vi "Book Picture - p24_h2e.vi"() -> ()   [LabVIEW 2013]
uses:
  <vilib>/Analysis/baseanly.llb/Real A x B.vi
  <vilib>/Analysis/baseanly.llb/Real Inverse Matrix.vi
  <vilib>/Analysis/NI_AALBase.lvlib
panel:
  out "Y1":dbl=1.7320508075688776 format="%#_5g"
  out "X1":dbl=1.7320508075688776 format="%#_5g"
  # "Coodinate Reference System"
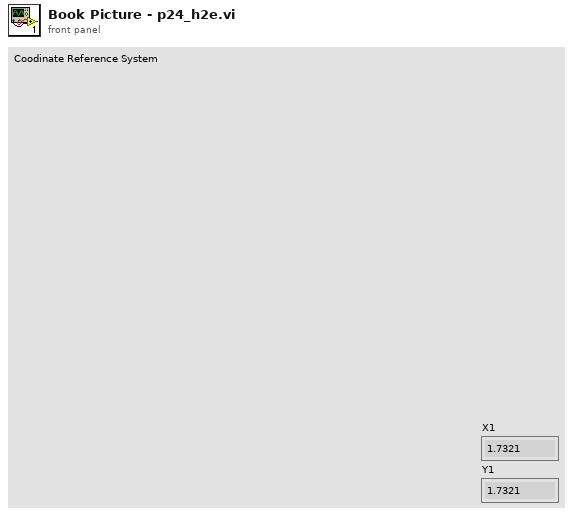
[diagram p1: front panel]
types:
  T1 = typedef "NI_Matrix.lvlib/RealMatrix.ctl" = dbl[][]
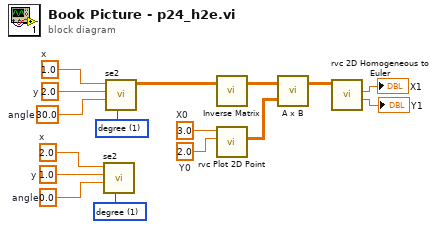
[diagram p0: block diagram]
diagram:
  w11 = 2.0  # Y0
  w12 = 3.0  # X0
  w3 = 0.0  # angle
  w2 = 1.0  # y
  w1 = 2.0  # x
  w4 = u16 1 items=["radians", "degree"] ("angle unit")
  w14 = 30.0  # angle
  w15 = 2.0  # y
  w16 = 1.0  # x
  w13 = u16 1 items=["radians", "degree"] ("angle unit")
  n1 = call "se2.vi"("angle unit"=w4, "theta"=w3, "y"=w2, "x"=w1) -> ()  [unwired: 6 in, 2 out]
  n2 = call "se2.vi"("angle unit"=w13, "theta"=w14, "y"=w15, "x"=w16) -> ("T"=w9:dbl[][])  [unwired: 6 in, 1 out]
  n3 = call-poly <vilib>:"Inverse Matrix.vi"("Input Matrix"=w9) -> ("Inverse Matrix"=w10:T1)  [unwired: 1 in, 1 out]
  n4 = call "rvc Plot 2D Point.vi"("Y"=w11, "X"=w12) -> ("Column vector"=w8:dbl[][])  [unwired: 8 in, 1 out]
  n5 = call-poly <vilib>:"A x B.vi"("B"=w8, "A"=w10) -> ("A x B"=w7:T1)  [unwired: 1 out]
  n6 = call "rvc 2D Homogeneous to Euler.vi"("T"=w7) -> ("y"=→"Y1":dbl, "x"=→"X1":dbl)  [unwired: 7 in, 2 out]
